vi "Configure Correction Spot.vi"(5 "Reference Value B (0.0)":dbl, 6 "Spot Frequency (20 Hz)":dbl=20.0, 7 "Reference Value A (0.0)":dbl, 8 "error in (no error)":errorcluster, 9 "Spot State (F:Disable)":bool, 10 "Spot No. (1)":i32=1, 11 "VISA resource name":refnum<visa-resource-name>) -> (0 "error out":errorcluster, 3 "VISA resource name out":refnum<visa-resource-name>)   [LabVIEW 2017, in "Agilent E4980.lvlib"]
doc: "Configures correction based on specified frequency point."
uses:
  Agilent E4980.lvlib
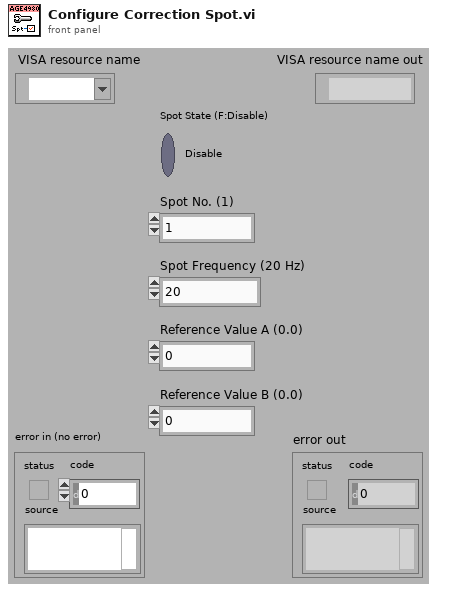
[diagram p1: front panel]
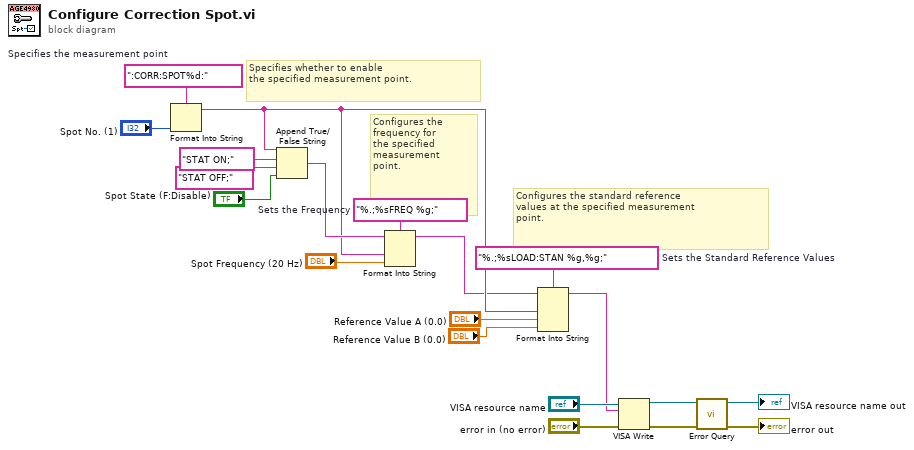
[diagram p0: block diagram]
diagram:
  w15 = "%.;%sLOAD:STAN %g,%g;"  # Sets the Standard Reference Values
  w16 = "%.;%sFREQ %g;"  # Sets the Frequency
  w20 = ":CORR:SPOT%d:"  # Specifies the measurement point
  # "Configures the standard reference\nvalues at the specified measurement\npoint."
  # "Configures the\nfrequency for\nthe specified\nmeasurement\npoint."
  # "Specifies whether to enable\nthe specified measurement point."
  n1 = Format Into String(format string=w20, "Spot No. (1)") -> (resulting string=w4:string)  [unwired: 2 in, 1 out]
  n2 = Append True/False String(1:"Spot State (F:Disable)", 2:"STAT OFF;" ("false string"), 3:"STAT ON;", 4:w4) -> (0:w7:string)
  n3 = Format Into String(format string=w16, initial string=w7, w4, "Spot Frequency (20 Hz)") -> (resulting string=w3:string)  [unwired: 1 in, 1 out]
  n4 = Format Into String(format string=w15, initial string=w3, w4, "Reference Value A (0.0)", "Reference Value B (0.0)") -> (resulting string=w12:string)  [unwired: 1 in, 1 out]
  n5 = VISA Write(VISA resource name="VISA resource name", write buffer=w12, error in (no error)="error in (no error)") -> (VISA resource name out=w11:refnum<visa-resource-name>, error out=w10:errorcluster)  [unwired: 1 out]
  n6 = call "Error Query.vi"("error in (no error)"=w10, "VISA resource name"=w11) -> ("error out"=→"error out":errorcluster, "VISA resource name out"=→"VISA resource name out":refnum<visa-resource-name>)  [unwired: 6 in, 2 out]
